vi "get_strobe_profile.vi"(11 "LED CONTROLS":i32[](array[numeric])) -> (3 "STROBE PROFILE":i32[][](array[numeric]))   [LabVIEW 2013]
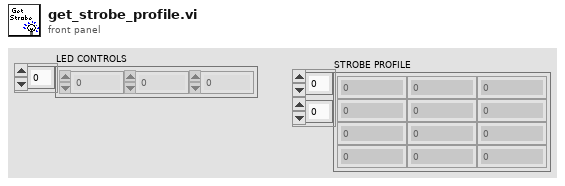
[diagram p1: front panel]
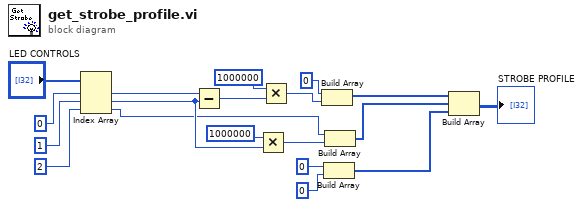
[diagram p0: block diagram]
diagram:
  n1 = Index Array(array="LED CONTROLS", index #1=0 ("index"), index #2=1 ("index"), index #3=2 ("index")) -> (element #1=w10:i32, element #2=w18:i32, element #3=w1:i32)
  n2 = Subtract(x=w10, y=w18) -> (x-y=w11:i32)
  n3 = Multiply(x=1000000, y=w18) -> (x*y=w3:i32)
  n4 = Multiply(x=1000000, y=w11) -> (x*y=w4:i32)
  n5 = Build Array(0 ("element"), w4) -> (w14:i32[])
  n6 = Build Array(0 ("index"), 0 ("index")) -> (w17:i32[])
  n7 = Build Array(w1, w3) -> (w19:i32[])
  n8 = Build Array(w14, w19, w17) -> (→"STROBE PROFILE":i32[][])
